vi "Config.vi"(8 "error in (no error)":errorcluster, 11 "MGI_Show Dialog in":refnum<class "MGI_Show Dialog.lvclass">) -> (0 "error out":errorcluster, 3 "MGI_Show Dialog out":refnum<class "MGI_Show Dialog.lvclass">)   [LabVIEW 2016, in "MGI_Show Dialog.lvclass"]
doc: "Authored by Derek E. Trepanier\nsupport@mooregoodideas.com\nwww.mooregoodideas.com\n\nCopyright (c) 2012, Moore Good Ideas, Inc.\n\nAll rights reserved.\n\nRedistribution and use in source and binary forms, with or without modification, are permitted provided that the following conditions are met:\n\n * Redistributions of source code must retain the above copyright notice, this list of conditions and the following disclaimer.\n * Redistributions in binary form must reproduce the above copyright notice, this list of conditions and the following disclaimer in the documentation and/or other materials provided with the distribution.\n * Neither the name of Moore Good Ideas, Inc. nor the names of its contributors may be used to endorse or promote products derived from this software without specific prior written permission.\n\nTHIS SOFTWARE IS PROVIDED BY THE COPYRIGHT HOLDERS AND CONTRIBUTORS \"AS IS\" AND ANY EXPRESS OR IMPLIED WARRANTIES, INCLUDING, BUT NOT LIMITED TO, THE IMPLIED WARRANTIES OF MERCHANTABILITY AND FITNESS FOR A PARTICULAR PURPOSE ARE DISCLAIMED. IN NO EVENT SHALL THE COPYRIGHT OWNER OR CONTRIBUTORS BE LIABLE FOR ANY DIRECT, INDIRECT, INCIDENTAL, SPECIAL, EXEMPLARY, OR CONSEQUENTIAL DAMAGES (INCLUDING, BUT NOT LIMITED TO, PROCUREMENT OF SUBSTITUTE GOODS OR SERVICES; LOSS OF USE, DATA, OR PROFITS; OR BUSINESS INTERRUPTION) HOWEVER CAUSED AND ON ANY THEORY OF LIABILITY, WHETHER IN CONTRACT, STRICT LIABILITY, OR TORT (INCLUDING NEGLIGENCE OR OTHERWISE) ARISING IN ANY WAY OUT OF THE USE OF THIS SOFTWARE, EVEN IF ADVISED OF THE POSSIBILITY OF SUCH DAMAGE."
uses:
  <userlib>/_MGI/Menu Building/Example/Plugin/Show Dialog/MGI_Show Dialog.lvclass
  <userlib>/_MGI/Menu Building/Example/Plugin/Show Dialog/MGI_Show Dialog.lvclass/MGI_Show Dialog.ctl
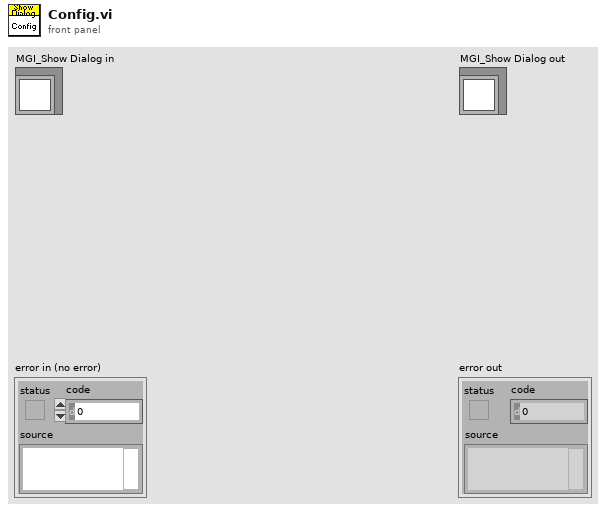
[diagram p1: front panel]
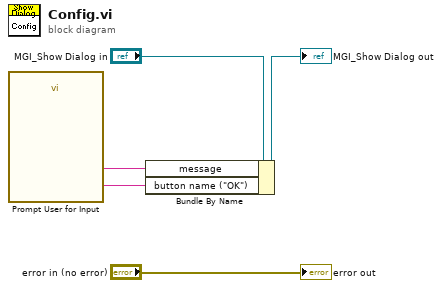
[diagram p0: block diagram]
diagram:
  n1 = call "Prompt User for Input"() -> ("Button Text"=w1:string, "Message"=w2:string)  [unwired: 16 in, 2 out]
  n2 = Bundle By Name(cluster="MGI_Show Dialog in", "message"=w2, "button name (\"OK\")"=w1) -> (→"MGI_Show Dialog out":refnum<class "MGI_Show Dialog.lvclass">)
  "error out" <- "error in (no error)"
